vi "advanced - RX (Chrono-Monitor) - SingleStandard-ReadFixedNumber.vi"() -> ()   [LabVIEW 2020]
uses:
  src/AIM664LV.lvlib
  src/_polimorphicInstances/session/Fdx Close Session (Port).vi
  src/_polimorphicInstances/session/Fdx Create Session (RX-Monitor).vi
  src/_polimorphicInstances/control/Fdx Stop (Rx).vi
  src/_polimorphicInstances/control/Fdx Start (Rx).vi
  src/_controls/session_monitor_config.ctl
  src/_controls/monitor_becw_type.ctl
  src/_controls/monitor_fhw0_type.ctl
  src/_controls/monitor_fhw1_type.ctl
  src/_controls/monitor_entrySize_type.ctl
  src/_controls/monitor_fhInfol_type.ctl
panel:
  in  "PortMap":u32
  out "conversion time uS":u32
  out "FrameHeaderInfo":T1 {"FHW0"."MacID" format="%03b"}
  out "Payload":u8[](array[numeric]) format="%.0x"
  out "BECW":T5
  out "IrigTime":T6
  out "EntryRead":u32
  out "BytesRead":u32
  in  "millisecond multiple":u32=100
  out "valuable data":i32
  in  "VLFilter":T7 {"FilterMode" items=["FDX_RX_VL_FLT_DIS", "FDX_RX_VL_FLT_ENA ", "FDX_RX_VL_FLT_ENA_INV"]; "VerificationMode" items=["FDX_RX_VL_CHECK_ENA_DEFAULT"=65535, "FDX_RX_VL_CHECK_REDMAM"=16, "DX_RX_VL_CHECK_TRAFIC"=8, "FDX_RX_VL_CHECK_FRAMESIZE"=4, "FDX_RX_VL_CHECK_SNINTEG"=2, "FDX_RX_VL_CHECK_INVPAC"=1, "FDX_RX_VL_CHECK_DISA"=0]; "PayloadMode" items=["FDX_PAYLOAD_FULL", "FDX_PAYLOAD_IP_EXT", "FDX_PAYLOAD_IP", "FDX_PAYLOAD_MAC"]; "EnableMode" items=["FDX_RX_VL_DIS "=0, "FDX_RX_VL_ENA_STAT"=1, "FDX_RX_VL_ENA_CNT "=2, "FDX_RX_VL_ENA_MON_ALL"=3, "FDX_RX_VL_ENA_MON_GOOD"=7, "FDX_RX_VL_ENA_EXT"=4]}
  in  "MaxFileSize MB (1)":u32=1
  out "error out":errorcluster
  in  "MonCapMode":T8 {"Strobe" items=["FDX_MON_STROBE_DIS", "FDX_MON_STROBE_STOP", "FDX_MON_STROBE_START"]; "CaptureMode" items=["FDX_MON_SINGLE ", "FDX_MON_CONTINUOUS", "FDX_MON_SELECTIVE", "FDX_MON_RECORDING", "FDX_MON_REROS", "FDX_MON_HMU"]}
  in  "EntryCount (1)":u32=1
  in  "ReadQualifier (0:full)":u32
  in  "MaxReadBytes":u32=65536
  out "QueueReadOut":T9
  out "QueueStatus":T10 {"QueueStatus" items=["FDX_MON_STAT_EMPTY", "FDX_MON_STAT_ FILLED", "FDX_MON_STAT_ FULL", "FDX_MON_STAT_ OVERFLOW", "FDX_MON_STAT_ ERROR"]}
  out "GlobMonSize":u32
  in  "RecordingFileName":path
  out "PortInitOut":T11 {"PortConfig" items=["FDX_SINGLE", "FDX_REDUNDANT"]}
  out "GlbMonBufferSizeOut":u32
  in  "Board":u32
  in  "Port":u32=1
  in  "DefaultPayloadMode (Full)":u32(ring) items=["FDX_PAYLOAD_FULL", "FDX_PAYLOAD_IP_EXT", "FDX_PAYLOAD_IP", "FDX_PAYLOAD_MAC"]
  in  "MonitorConfig":T12={"DefaultCronoMode"=2, "GlbMonBufferSizeIn"=0} {"DefaultCronoMode" items=["FDX_RX_DEFAULT_ENA_CNT", "FDX_RX_DEFAULT_MON_ENA_ALL", "FDX_RX_DEFAULT_MON_ENA_GOOD"]}
  in  "stop":bool
  out "current irig time":T13
  out "current time":timestamp
  out "read time uS":u32(graph)
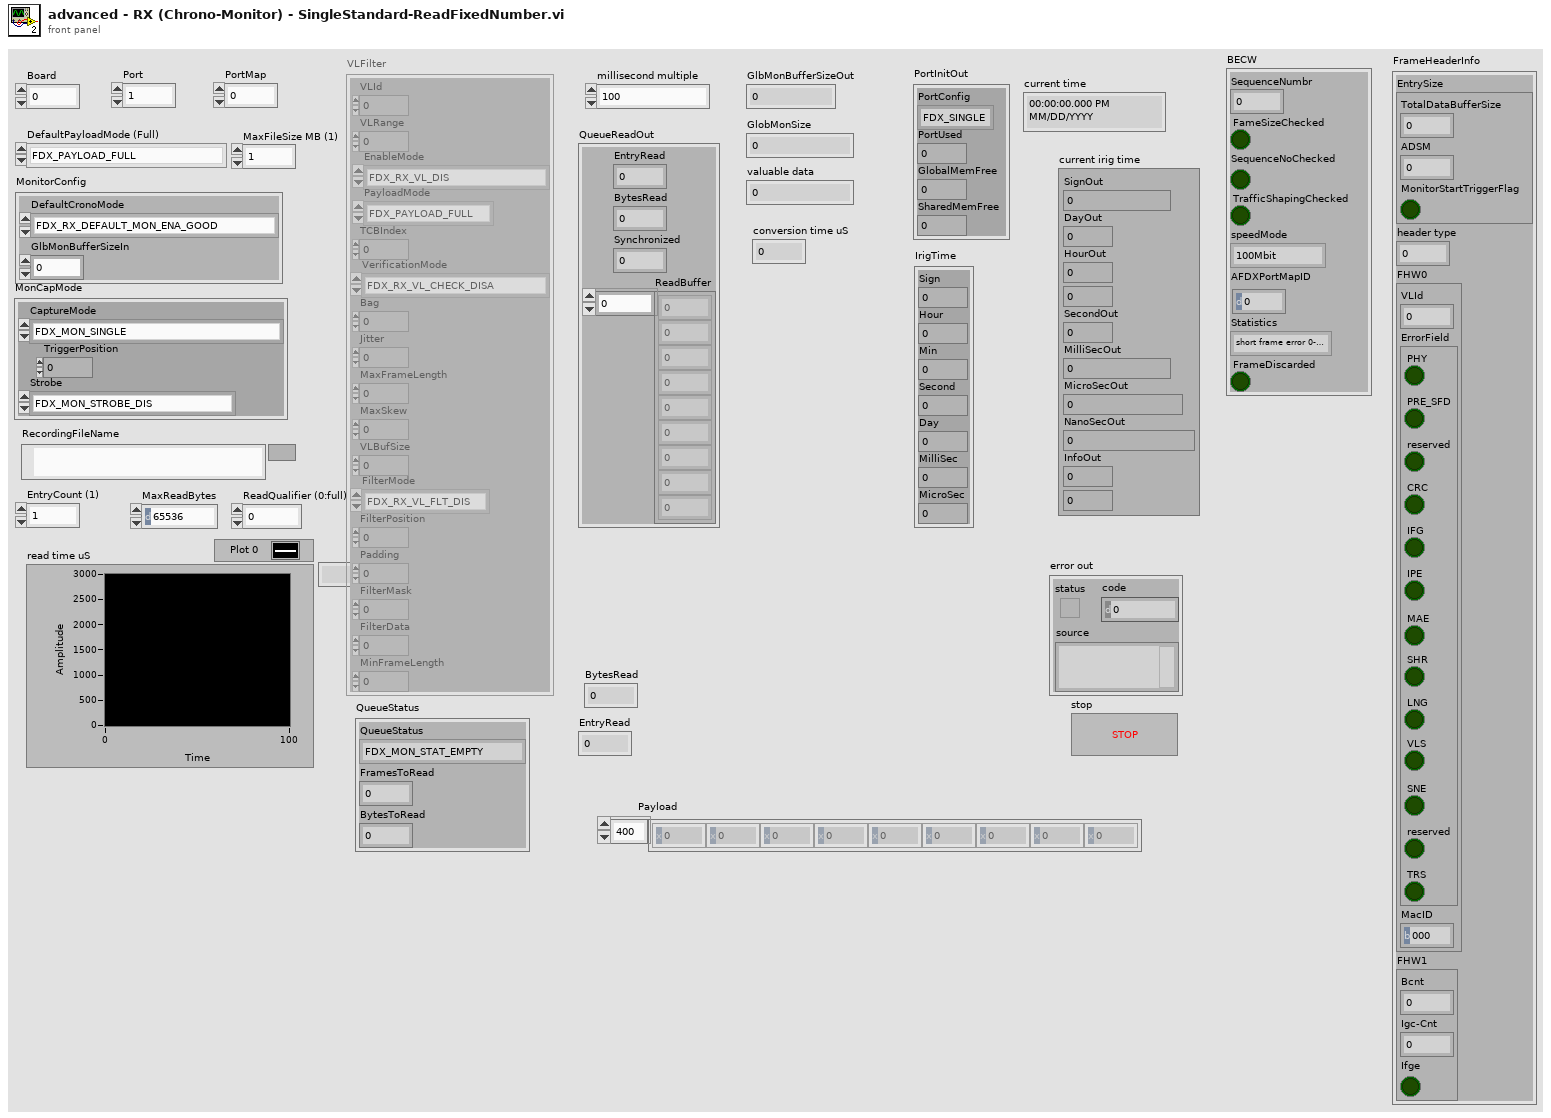
[diagram p1: front panel]
types:
  T1 = typedef "AIM664LV.lvlib/monitor_fhInfol_type.ctl" = cluster{"EntrySize":T2, "header type":u32, "FHW0":T3, "FHW1":T4}
  T2 = typedef "AIM664LV.lvlib/monitor_entrySize_type.ctl" = cluster{"TotalDataBufferSize":u16, "ADSM":u16, "MonitorStartTriggerFlag":bool}
  T3 = typedef "AIM664LV.lvlib/monitor_fhw0_type.ctl" = cluster{"VLId":u16, "ErrorField":cluster{"PHY":bool, "PRE_SFD":bool, "reserved":bool, "CRC":bool, "IFG":bool, "IPE":bool, "MAE":bool, "SHR":bool, "LNG":bool, "VLS":bool, "SNE":bool, "reserved":bool, "TRS":bool}, "MacID":u8}
  T4 = typedef "AIM664LV.lvlib/monitor_fhw1_type.ctl" = cluster{"Bcnt":u16, "Igc-Cnt":u16, "Ifge":bool}
  T5 = typedef "AIM664LV.lvlib/monitor_becw_type.ctl" = cluster{"SequenceNumbr":u8, "FameSizeChecked":bool, "SequenceNoChecked":bool, "TrafficShapingChecked":bool, "speedMode":enum16{"100Mbit", "10Mbit", "1Gbit"}, "AFDXPortMapID":u8, "Statistics":enum16{"short frame error 0-63Bytes", "64-127 Bytes", "128-255 Bytes", "256-511 Bytes", "512-1023 Bytes", "1024-1518 Bytes", ">1518 Bytes"}, "FrameDiscarded":bool}
  T6 = cluster{"Sign":i32, "Hour":u32, "Min":u32, "Second":u32, "Day":u32, "MilliSec":u32, "MicroSec":u32}
  T7 = cluster{"VLId":u32, "VLRange":u32, "EnableMode":u32, "PayloadMode":u32, "TCBIndex":u32, "VerificationMode":u32, "Bag":u32, "Jitter":u32, "MaxFrameLength":u32, "MaxSkew":u32, "VLBufSize":u32, "FilterMode":u32, "FilterPosition":u32, "Padding":u32, "FilterMask":u32, "FilterData":u32, "MinFrameLength":u32}
  T8 = cluster{"CaptureMode":u32, "TriggerPosition":u32, "Strobe":u32}
  T9 = cluster{"EntryRead":u32, "BytesRead":u32, "Synchronized":u32, "ReadBuffer":u8[]}
  T10 = cluster{"QueueStatus":u32, "FramesToRead":u32, "BytesToRead":u32}
  T11 = cluster{"PortConfig":u32, "PortUsed":u32, "GlobalMemFree":u32, "SharedMemFree":u32}
  T12 = typedef "AIM664LV.lvlib/session_monitor_config.ctl" = cluster{"DefaultCronoMode":u32, "GlbMonBufferSizeIn":u32}
  T13 = cluster{"SignOut":i32, "DayOut":u32, "HourOut":u32, "MinOut":u32, "SecondOut":u32, "MilliSecOut":u32, "MicroSecOut":u32, "NanoSecOut":u32, "InfoOut":u32, "Mode":u32}
  T14 = typedef "AIM664LV.lvlib/IrigTime.ctl" = cluster{"Sign":i32, "Day":u32, "Hour":u32, "Min":u32, "Second":u32, "MilliSec":u32, "MicroSec":u32}
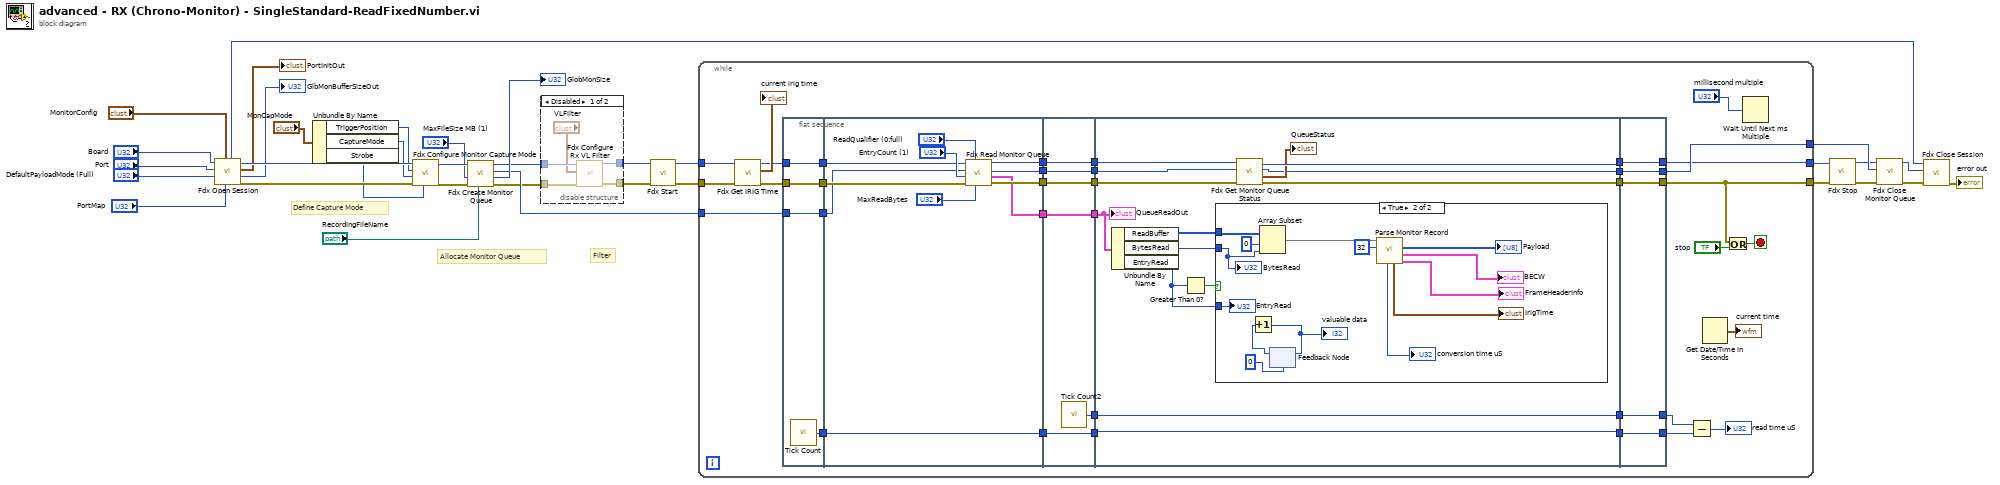
[diagram p0: block diagram]
diagram:
  # "Filter"
  # "Allocate Monitor Queue"
  # "Define Capture Mode"
  n1 = call-poly "Fdx Open Session.vi"("PortMap"="PortMap", "MonitorConfig"="MonitorConfig", "DefaultPayloadMode (Full)"="DefaultPayloadMode (Full)", "port"="Port", "board"="Board") -> ("error out"=w33:errorcluster, "GlbMonBufferSizeOut"=→"GlbMonBufferSizeOut":u32, "PortInitOut"=→"PortInitOut":T11, "InstrumentHandle_port out"=w34:u32, "InstrumentHandle_board out"=w1:u32)  [unwired: 1 in, 1 out]
  n2 = Unbundle By Name("MonCapMode") -> ("TriggerPosition"=w4:u32, "CaptureMode"=w3:u32, "Strobe"=w2:u32)
  n3 = call "Fdx Configure Monitor Capture Mode.vi"("Strobe"=w2, "error in (no error)"=w33, "CaptureMode"=w3, "TriggerPosition"=w4, "InstrumentHandle_port in"=w34) -> ("error out"=w31:errorcluster, "InstrumentHandle_port out"=w32:u32)  [unwired: 5 in]
  n4 = call "Fdx Create Monitor Queue.vi"("RecordingFileName"="RecordingFileName", "error in (no error)"=w31, "MaxFileSize MB (1)"="MaxFileSize MB (1)", "InstrumentHandle_port in"=w32) -> ("error out"=w14:errorcluster, "GlobMonSize"=→"GlobMonSize":u32, "QueueIdOut"=w20:u32, "InstrumentHandle_port out"=w15:u32)  [unwired: 4 in]
  n5 = disable-structure shown="Disabled" {
    disable-tunnel: w15 -> [w39 w41]
    disable-tunnel: w14 -> [w38 w40]
    disable-tunnel: [w37 w41] -> w13
    disable-tunnel: [w36 w40] -> w12
    frame Disabled {
      n6 = call "Fdx Configure Rx VL Filter.vi"("error in (no error)"=w38, "VLFilter"="VLFilter", "InstrumentHandle_port in"=w39) -> ("error out"=w36:errorcluster, "InstrumentHandle_port out"=w37:u32)  [unwired: 7 in]
    }
    frame Enabled {
    }
  }
  n7 = call-poly "Fdx Start.vi"("error in (no error)"=w12, "InstrumentHandle_port in"=w13) -> ("error out"=w23:errorcluster, "InstrumentHandle_port out"=w24:u32)  [unwired: 8 in]
  n8 = while {
    tunnel: [w42] -> w25
    tunnel: w24 -> [w61]
    tunnel: w23 -> [w60]
    tunnel: w20 -> [w58]
    tunnel: [w51] -> w17
    tunnel: [w44] -> w8
    stop <- w76 stop-if-true
    n9 = call "Fdx Get IRIG Time.vi"("error in (no error)"=w60, "InstrumentHandle_board in"=w61) -> ("error out"=w73:errorcluster, "Curent Irig Time"=→"current irig time":T13, "InstrumentHandle_board out"=w45:u32)  [unwired: 7 in]
    n10 = flat-sequence {
      tunnel: w73 -> [w81]
      tunnel: [w81] -> w68
      tunnel: [w80] -> w67
      tunnel: [w79] -> w59
      tunnel: w58 -> [w79]
      tunnel: [w78] -> w46
      tunnel: w45 -> [w78]
      tunnel: w68 -> [w91]
      tunnel: w67 -> [w92]
      tunnel: [w92] -> w66
      tunnel: w59 -> [w83]
      tunnel: [w90] -> w56
      tunnel: [w89] -> w54
      tunnel: [w87] -> w49
      tunnel: [w86] -> w47
      tunnel: w46 -> [w82]
      tunnel: w66 -> [w98]
      tunnel: [w98] -> w65
      tunnel: [w97] -> w62
      tunnel: [w96] -> w57
      tunnel: w56 -> [w96]
      tunnel: [w95] -> w55
      tunnel: w54 -> [w95]
      tunnel: [w94] -> w50
      tunnel: w49 -> [w94]
      tunnel: [w93] -> w48
      tunnel: w47 -> [w93]
      tunnel: w65 -> [w112]
      tunnel: [w112] -> w70
      tunnel: [w111] -> w63
      tunnel: w62 -> [w111]
      tunnel: w57 -> [w110]
      tunnel: w55 -> [w109]
      tunnel: [w108] -> w53
      tunnel: [w107] -> w52
      tunnel: w50 -> [w105]
      tunnel: w48 -> [w100]
      tunnel: [w99] -> w43
      tunnel: [w131] -> w71
      tunnel: w70 -> [w131]
      tunnel: [w130] -> w64
      tunnel: w63 -> [w130]
      tunnel: [w129] -> w42
      tunnel: w53 -> [w129]
      tunnel: [w128] -> w51
      tunnel: w52 -> [w128]
      tunnel: [w127] -> w44
      tunnel: w43 -> [w127]
      frame #0 {
        n11 = call "Tick Count"() -> ("Tick Count(uSec)"=w80:u32)
      }
      frame #1 {
        n12 = call "Fdx Read Monitor Queue.vi"("MaxReadBytes"="MaxReadBytes", "ReadQualifier (0:full)"="ReadQualifier (0:full)", "error in (no error)"=w91, "EntryCount (1)"="EntryCount (1)", "QueueId in"=w83, "InstrumentHandle_port in"=w82) -> ("error out"=w89:errorcluster, "QueueReadOut"=w87:T9, "QueueId out"=w86:u32, "InstrumentHandle_port out"=w90:u32)  [unwired: 2 in]
      }
      frame #2 {
        n13 = call "Tick Count2"() -> ("Tick Count(uSec)"=w97:u32)
      }
      frame #3 {
        n14 = Unbundle By Name(w105) -> ("ReadBuffer"=w103:u8[], "BytesRead"=w102:u32, "EntryRead"=w101:u32)
        n15 = Greater Than 0?(x=w101) -> (x > 0?=w104:bool)
        n16 = case shown="True" w104 {
          tunnel: w103 -> [_ w123]
          tunnel: w102 -> [_ w121]
          tunnel: w101 -> [_ w120]
          frame False {
          }
          frame True {
            n17 = Array Subset(array=w123, index=0, length=w121) -> (w117:u8[])
            n18 = feedback #1(0) -> (w126:i32)
            n19 = Increment(x=w126) -> (x+1=w125:i32)
            "valuable data" <- w125
            n20 = feedback-in #1(w125) -> ()
            n21 = call "Parse Monitor Record.vi"("header size bytes (32)"=32 ("header size bytes (36)"), "Record In"=w117) -> ("FrameHeaderInfo"=→"FrameHeaderInfo":T1, "BECW"=→"BECW":T5, "Payload"=→"Payload":u8[], "IrigTime"=→"IrigTime":T14, "conversion time uS"=→"conversion time uS":u32)  [unwired: 4 in, 1 out]
            "BytesRead" <- w121
            "EntryRead" <- w120
          }
        }
        n22 = call "Fdx Get Monitor Queue Status.vi"("error in (no error)"=w109, "QueueId in"=w100, "InstrumentHandle_port in"=w110) -> ("error out"=w107:errorcluster, "QueueStatus"=→"QueueStatus":T10, "QueueId out"=w99:u32, "InstrumentHandle_port out"=w108:u32)  [unwired: 5 in]
        "QueueReadOut" <- w105
      }
      frame #4 {
      }
    }
    n23 = Subtract(x=w64, y=w71) -> (x-y=→"read time uS":u32)
    n24 = Get Date/Time In Seconds() -> (seconds since 1Jan1904=→"current time":timestamp)
    n25 = Or(x=w51, y="stop") -> (x .or. y?=w76:bool)
    n26 = Wait Until Next ms Multiple(millisecond multiple="millisecond multiple") -> ()  [unwired: 1 out]
  }
  n27 = call-poly "Fdx Stop.vi"("error in (no error)"=w17, "InstrumentHandle_port in"=w25) -> ("error out"=w19:errorcluster, "InstrumentHandle_port out"=w7:u32)  [unwired: 8 in]
  n28 = call "Fdx Close Monitor Queue.vi"("error in (no error)"=w19, "QueueId"=w8, "InstrumentHandle_port in"=w7) -> ("error out"=w18:errorcluster, "InstrumentHandle_port out"=w6:u32)  [unwired: 7 in]
  n29 = call-poly "Fdx Close Session.vi"("error in (no error)"=w18, "InstrumentHandle_port in"=w6, "InstrumentHandle_board in"=w1) -> ("error out"=→"error out":errorcluster)  [unwired: 8 in]
